vi "viewerTestDataGenerator.vi"   [LabVIEW 2011, in "viewer.lvclass"]
uses:
  Pollers/ttm_poller_panel_class/viewer.lvclass
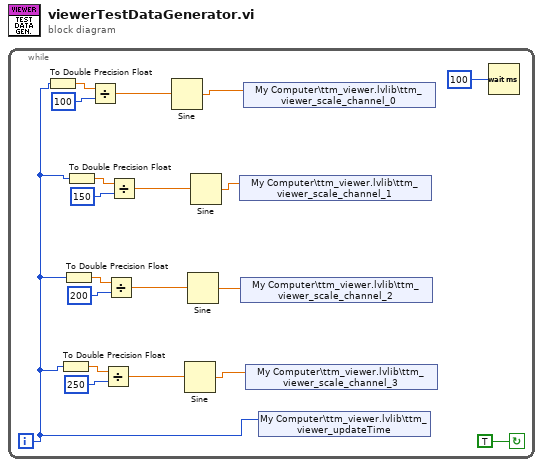
[diagram p0: block diagram]
diagram:
  n1 = while {
    i -> [w1]
    stop <- TRUE continue-if-true
    n2 = To Double Precision Float(number=w1) -> (double precision float=w15:dbl)
    n3 = To Double Precision Float(number=w1) -> (double precision float=w5:dbl)
    n4 = To Double Precision Float(number=w1) -> (double precision float=w8:dbl)
    n5 = To Double Precision Float(number=w1) -> (double precision float=w11:dbl)
    n6 = Divide(x=w15, y=100) -> (x/y=w16:dbl)
    n7 = Divide(x=w5, y=250) -> (x/y=w6:dbl)
    n8 = Divide(x=w8, y=200) -> (x/y=w9:dbl)
    n9 = Divide(x=w11, y=150) -> (x/y=w12:dbl)
    n10 = Sine(x=w16) -> (sin(x)=w18:dbl)
    n11 = Sine(x=w6) -> (sin(x)=w2:dbl)
    n12 = Sine(x=w9) -> (sin(x)=w3:dbl)
    n13 = Sine(x=w12) -> (sin(x)=w4:dbl)
    n14 = shared-variable "My Computer\\ttm_viewer.lvlib\\ttm_viewer_scale_channel_1"(w4) -> ()  [unwired: 1 in, 1 out]
    n15 = shared-variable "My Computer\\ttm_viewer.lvlib\\ttm_viewer_scale_channel_2"(w3) -> ()  [unwired: 1 in, 1 out]
    n16 = shared-variable "My Computer\\ttm_viewer.lvlib\\ttm_viewer_scale_channel_0"(w18) -> ()  [unwired: 1 in, 1 out]
    n17 = shared-variable "My Computer\\ttm_viewer.lvlib\\ttm_viewer_scale_channel_3"(w2) -> ()  [unwired: 1 in, 1 out]
    n18 = shared-variable "My Computer\\ttm_viewer.lvlib\\ttm_viewer_updateTime"(w1) -> ()  [unwired: 1 in, 1 out]
    n19 = Wait (ms)(milliseconds to wait=u32 100) -> ()  [unwired: 1 out]
  }
